vi "STM Set Meta Data (Serial Ref).vi"(7 "Meta data":T1[](array[typedef]), 8 "error in":errorcluster, 11 "VISA resource name":refnum<visa-resource-name>) -> (0 "error out":errorcluster, 3 "Connection Info Out":T2)   [LabVIEW 2014, in "QwaveSys Raspberry Pi Library.lvlib"]
doc: "Assigns the meta data cluster associated with this STM session."
uses:
  QwaveSys Raspberry Pi Library.lvlib
  stm_Serial Connection Info.ctl
  _SubVIs/stm_MetaDataElement.ctl
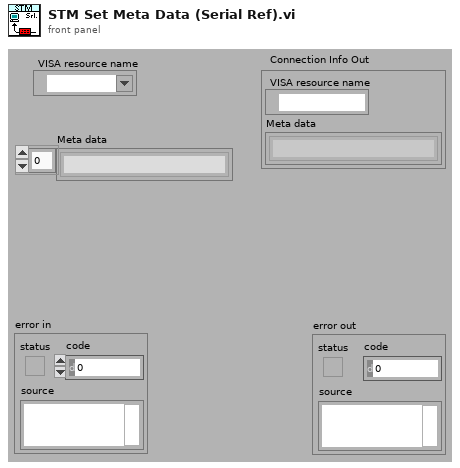
[diagram p1: front panel]
types:
  T1 = typedef "QwaveSys Raspberry Pi Library.lvlib/stm_MetaDataElement.ctl" = string
  T2 = typedef "QwaveSys Raspberry Pi Library.lvlib/stm_Serial Connection Info.ctl" = cluster{"VISA resource name":refnum<visa-resource-name>, "Meta data":T1[]}
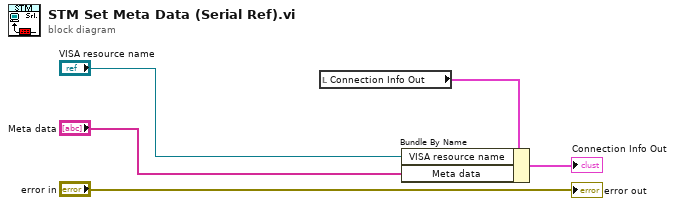
[diagram p0: block diagram]
diagram:
  n1 = local read "Connection Info Out"() -> (w1:T2)
  n2 = Bundle By Name(cluster=w1, "VISA resource name"="VISA resource name", "Meta data"="Meta data") -> (→"Connection Info Out":T2)
  "error out" <- "error in"
